vi "Read Spec Page Path.vi"(8 "error in (no error)":errorcluster, 11 "MeasurementMetaData in":refnum<class "MeasurementMetaData.lvclass">) -> (0 "error out":errorcluster, 2 "Path to Spec Page VI":path, 3 "MeasurementMetaData out":refnum<class "MeasurementMetaData.lvclass">)   [LabVIEW 2013, in "MeasurementMetaData.lvclass"]
uses:
  MeasurementMetaData.lvclass
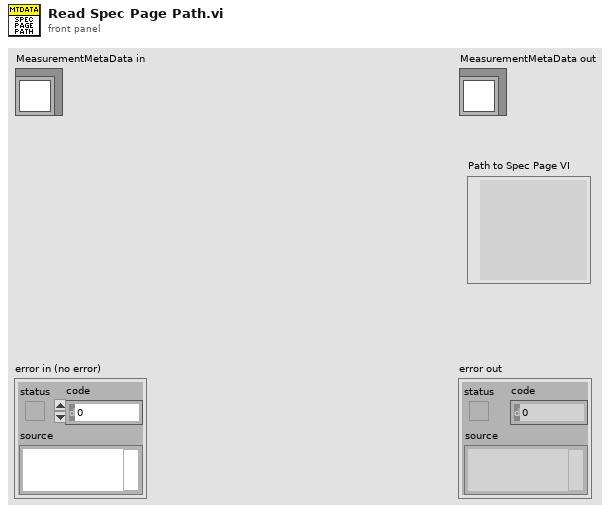
[diagram p1: front panel]
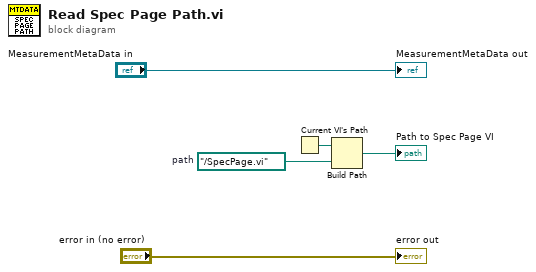
[diagram p0: block diagram]
diagram:
  w2 = path "../SpecPage.vi"  # path
  n1 = Current VI's Path() -> (path=w3:path)
  n2 = Build Path(base path=w3, name or relative path=w2) -> (appended path=→"Path to Spec Page VI":path)
  "error out" <- "error in (no error)"
  "MeasurementMetaData out" <- "MeasurementMetaData in"
